vi "Encoded String To UTF-8.vi"(8 "error in (no error)":errorcluster, 10 "Encoded string":string, 11 "Encoding in":refnum<class "CConfig Encoding.lvclass">) -> (0 "error out":errorcluster, 2 "UTF-8 string":string, 3 "Encoding out":refnum<class "CConfig Encoding.lvclass">)   [LabVIEW 2013, in "CConfig Encoding.lvclass"]
doc: "Copyright 2018, Carya Automatisering, Wiebe Walstra."
uses:
  CConfig Encoding.lvclass
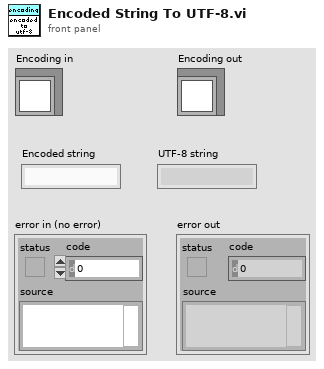
[diagram p1: front panel]
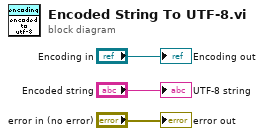
[diagram p0: block diagram]
diagram:
  "error out" <- "error in (no error)"
  "Encoding out" <- "Encoding in"
  "UTF-8 string" <- "Encoded string"
